vi "TransformObjectPosition_Objects.vi"(4 "Pixel size Y":dbl, 6 "Image time":dbl, 8 "error in (no error)":errorcluster, 9 "Pixel size X":dbl, 10 "Objects":T1(array[cluster]) {"Aspect Ratio" format="%.2f"; "Orientation" format="%.2f"; "Area" format="%.2f"; "Object Center"."Y" format="%.2f"; "Object Center"."X" format="%.2f"}, 11 "Spacetime cluster":T2) -> (0 "error out":errorcluster, 1 "Focus out":dbl, 2 "Y out":dbl, 3 "X out":dbl)   [LabVIEW 2012]
panel:
  out "Y center":dbl(graph)
  out "X center":dbl(graph)
  out "X stage":dbl(graph)
  out "Y stage":dbl(graph)
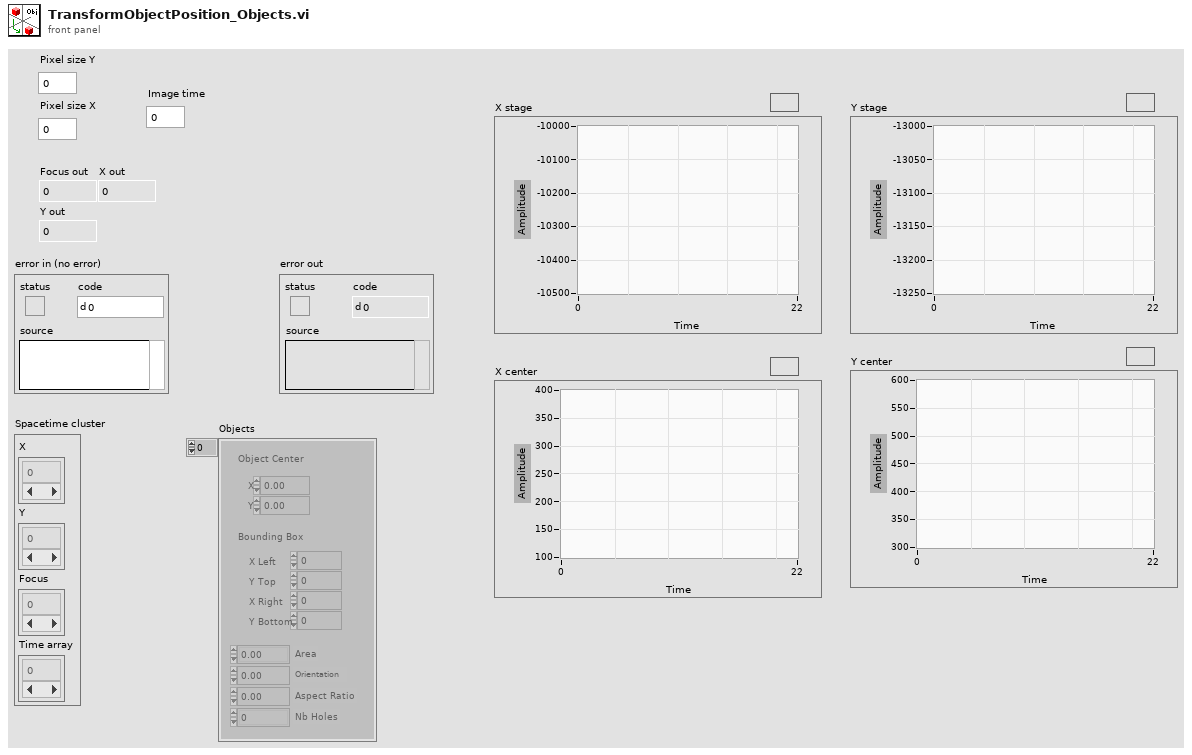
[diagram p1: front panel]
types:
  T1 = cluster{"Object Center":cluster{"X":sgl, "Y":sgl}, "Bounding Box":cluster{"X Left":i32, "Y Top":i32, "X Right":i32, "Y Bottom":i32}, "Area":sgl, "Orientation":sgl, "Aspect Ratio":sgl, "Nb Holes":i32}[]
  T2 = cluster{"X":dbl[], "Y":dbl[], "Focus":dbl[], "Time array":dbl[]}
  T3 = cluster{"Object Center":cluster{"X":sgl, "Y":sgl}, "Bounding Box":cluster{"X Left":i32, "Y Top":i32, "X Right":i32, "Y Bottom":i32}, "Area":sgl, "Orientation":sgl, "Aspect Ratio":sgl, "Nb Holes":i32}
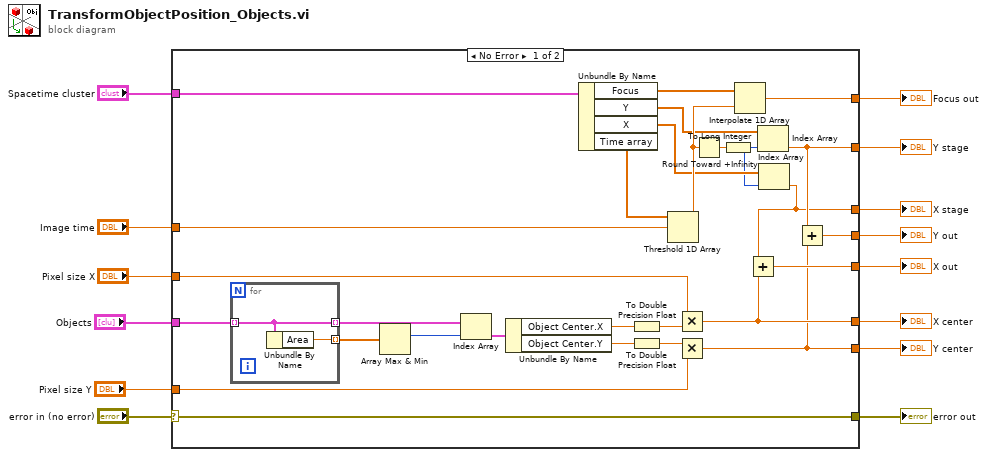
[diagram p0: block diagram]
diagram:
  n1 = case shown="No Error" "error in (no error)" {
    selector: "error in (no error)" -> [w36 w45]
    tunnel: [w36 w45] -> w13
    tunnel: "Objects" -> [w18 _]
    tunnel: "Pixel size X" -> [w41 _]
    tunnel: "Image time" -> [w40 _]
    tunnel: [w39 _] -> w10
    tunnel: [w38 _] -> w9
    tunnel: [w37 _] -> w8
    tunnel: "Spacetime cluster" -> [w35 _]
    tunnel: [w29 _] -> w6
    tunnel: [w26 _] -> w5
    tunnel: [w24 _] -> w4
    tunnel: [w23 _] -> w3
    tunnel: "Pixel size Y" -> [w21 _]
    frame No Error {
      n2 = for {
        tunnel: w18 -> [w43] mode=indexing
        tunnel: [w44] -> w16 mode=indexing
        tunnel: [w43] -> w17 mode=indexing
        n3 = Unbundle By Name(w43) -> ("Area"=w44:sgl)
      }
      n4 = Array Max & Min(array=w16) -> (max index (indices)=w15:i32)  [unwired: 3 out]
      n5 = Index Array(array=w17, index=w15) -> (element=w42:T3)
      n6 = Unbundle By Name(w42) -> ("Object Center.X"=w25:sgl, "Object Center.Y"=w22:sgl)
      n7 = Unbundle By Name(w35) -> ("Focus"=w34:dbl[], "Y"=w30:dbl[], "X"=w28:dbl[], "Time array"=w33:dbl[])
      n8 = To Double Precision Float(number=w25) -> (double precision float=w20:dbl)
      n9 = To Double Precision Float(number=w22) -> (double precision float=w19:dbl)
      n10 = Threshold 1D Array(2:w40, 3:w33) -> (0:w32:dbl)  [unwired: 1 in]
      n11 = Multiply(x=w41, y=w20) -> (x*y=w24:dbl)
      n12 = Multiply(x=w19, y=w21) -> (x*y=w23:dbl)
      n13 = Round Toward +Infinity(x=w32) -> (ceil(x): smallest int >= x=w31:dbl)
      n14 = To Long Integer(number=w31) -> (32bit integer=w27:i32)
      n15 = Interpolate 1D Array(1:w32, 2:w34) -> (0:w39:dbl)
      n16 = Index Array(array=w30, index=w27) -> (element=w29:dbl)
      n17 = Index Array(array=w28, index=w27) -> (element=w26:dbl)
      n18 = Add(x=w26, y=w24) -> (x+y=w37:dbl)
      n19 = Add(x=w29, y=w23) -> (x+y=w38:dbl)
    }
    frame Error {
    }
  }
  "error out" <- w13
  "Focus out" <- w10
  "Y out" <- w9
  "X out" <- w8
  "Y stage" <- w6
  "X stage" <- w5
  "X center" <- w4
  "Y center" <- w3
